vi "WaterFall.vi"() -> ()   [LabVIEW 2014]
uses:
  <vilib>/Simulation/Scripting/Companion Diagram/SimConfigNode/SimParams.ctl
  <vilib>/Simulation/Scripting/Companion Diagram/SimConfigNode/_simSolvers.ctl
  <vilib>/Simulation/Implementation/Shared/SIMSCR Execution Mode.ctl
  <vilib>/Simulation/Param Hierarchy/Typedefs/SIMPH Param Control Actions.ctl
  <vilib>/Simulation/Implementation/Shared/SIM limit type.ctl
  <vilib>/Simulation/Implementation/Shared/NILVSim_ParamChanged.vi
  <vilib>/Simulation/Implementation/Shared/NILVSIM_BeginStep.vi
  <vilib>/Simulation/DataSources/Implementation/NILVSim Step.llb/SIM Step (scalar).vi
  <vilib>/Simulation/Nonlinear/Implementation/NILVSim Switch.llb/SIM Switch (scalar).vi
  <vilib>/Simulation/DataSources/Implementation/NILVSim Pulse Generator.llb/SIM Pulse Generator (scalar).vi
  <vilib>/Simulation/ContinuousLinear/Implementation/NILVSim Transfer Function.llb/SIM Transfer Function Distributor (SISO).vi
  <vilib>/Simulation/ContinuousLinear/Implementation/NILVSim Integrator new.llb/SIM Integrator distributor (scalar).vi
  <vilib>/Simulation/ContinuousLinear/Implementation/NILVSim Derivative.llb/SIM derivative (scalar).vi
  <vilib>/Simulation/Nonlinear/Implementation/NILVSim Saturation.llb/SIM Saturation (scalar).vi
  <vilib>/Simulation/ContinuousLinear/Implementation/NILVSim Transport Delay.llb/SIM Transport Delay Distributor (scalar).vi
  <vilib>/Simulation/ContinuousLinear/Implementation/NILVSim Transport Delay.llb/SIM Transport Delay Collector (scalar).vi
  <vilib>/Simulation/ContinuousLinear/Implementation/NILVSim Integrator new.llb/SIM Integrator collector (scalar).vi
  <vilib>/Simulation/SignalDisplay/Implementation/NILVSim Time Waveform.llb/SIM Time Waveform (vector).vi
  <vilib>/Simulation/ContinuousLinear/Implementation/NILVSim Transfer Function.llb/SIM Transfer Function Collector (SISO).vi
  <vilib>/Simulation/Implementation/Shared/NILVSim_Manager.vi
  <vilib>/Utility/error.llb/Clear Errors.vi
  <vilib>/Simulation/Implementation/Shared/NILVSim_FinalizeModel.vi
  <vilib>/Simulation/Implementation/Shared/SIM Unbundle Sim Info.vi
  <vilib>/Simulation/Implementation/Shared/NILVSim_Initialize.vi
  <vilib>/Simulation/Utility/Implementation/NILVSim Get Time and IsAcceptedStep.vi
  <vilib>/Simulation/Implementation/Shared/SIMSH Read Queue.vi
  <vilib>/Simulation/Implementation/Shared/NILVSim_GetModelError.vi
  <vilib>/Simulation/Implementation/Shared/SIM Bundle Sim Info.vi
  <vilib>/Simulation/Scripting/Companion Diagram/SimConfigNode/SimDog.xnode
  <vilib>/Simulation/Implementation/XNodeFramework/SimXNode/SimX.xnode
  <vilib>/Simulation/ContinuousLinear/Implementation/NILVSim Integrator new.llb/SIM Integrator (scalar).vi
  <vilib>/Simulation/ContinuousLinear/Implementation/NILVSim Transport Delay.llb/SIM Transport Delay Indirect (scalar).vi
  <vilib>/Simulation/ContinuousLinear/Implementation/NILVSim Transfer Function.llb/SIM Transfer Function (SISO).vi
  <vilib>/Simulation/Implementation/Shared/NI_SIM_Implementation.lvlib
panel:
  in  "F1_0 2":dbl=1.0
  out "X 0":dbl caption="ISE 2"
  in  "tpm":dbl
  in  "Ttm":dbl
  in  "Kpm":dbl
  in  "Ks":dbl
  in  "tps":dbl
  out "Kcs":dbl
  out "Tis":dbl
  out "Kcm":dbl
  out "Tim":dbl
  out "Tdm":dbl
  in  "Incremento P1\nAmplitud":dbl=0.05
  out "DP1 Perturbacion":dbl caption="ISE 2"
  in  "Incremento P1\nduracion":dbl=10.0
  in  "Retardo en la \ntuberia":dbl=3.0
  in  "Fd Duraci—n\n perturbaci—n":dbl=10.0
  in  "1=ZN, 0=AMIGO":dbl
  out "Kc":dbl
  out "Ti":dbl
  out "Td":dbl
  in  "F1_0":dbl=1.0
  in  "H0":dbl=1.0
  in  "Href":dbl=1.0
  out "Fd Perturbacion":dbl caption="ISE 2"
  out "Tank  Cascade":dbl(slide) scale=0.0..4.0
  out "ISE 2":dbl
  out "ISE 1":dbl
  out "input flow":waveform(dbl)[](graph)
  in  "factor Kc":dbl=1.0
  in  "factor Td":dbl=1.0
  in  "Fd Amplitud\n perturbacion":dbl
  out "Td2":dbl
  out "Ti2":dbl
  out "Kc2":dbl
  out "Td1":dbl
  out "Ti1":dbl
  out "Kc1":dbl
  in  "tp":dbl=2.0
  in  "Tt":dbl=3.0
  in  "Kp":dbl=20.0
  out "ISE":waveform(dbl)[](graph)
  out "Tank B.R.C.":dbl(slide) scale=0.0..4.0
  in  "K1":dbl=1.0
  in  "A1":dbl=1.0
  in  "factor Ti":dbl=1.0
  out "Alturas":waveform(dbl)[](graph)
  # "Estudio del control en cascada"
  # "Altura de Referencia"
  # "PERTURBACIONES"
  # "SISTEMA"
  # "IDENTIFICACIÓN\nC.R.B."
  # "IDENTIF. \nESCLAVO"
  # "IDENTIF. \nMAESTRO"
  # "CONTROLADOR\nESCLAVO"
  # "CONTROLADOR\nMAESTRO"
  # "C.R.B"
  # "Z-N"
  # "AMIGO"
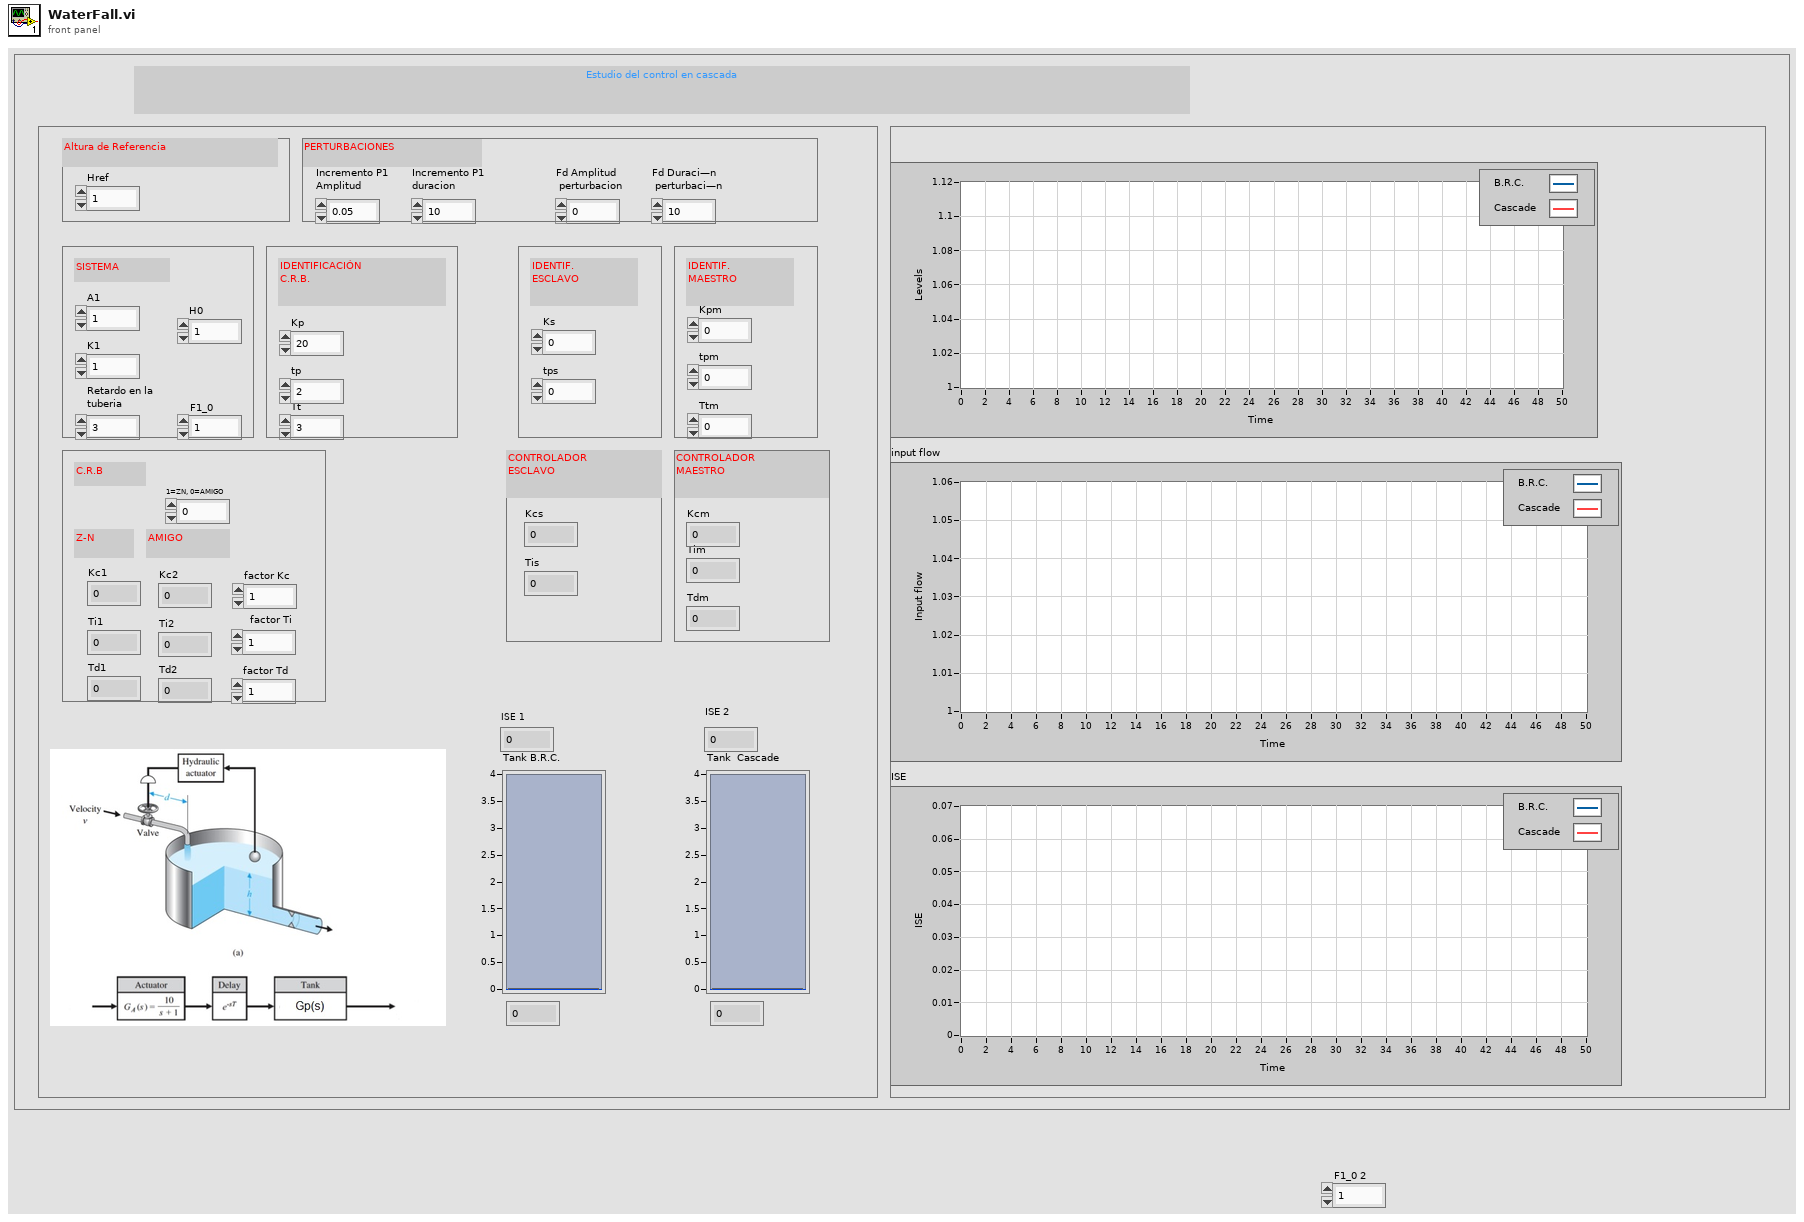
[diagram p1: front panel]
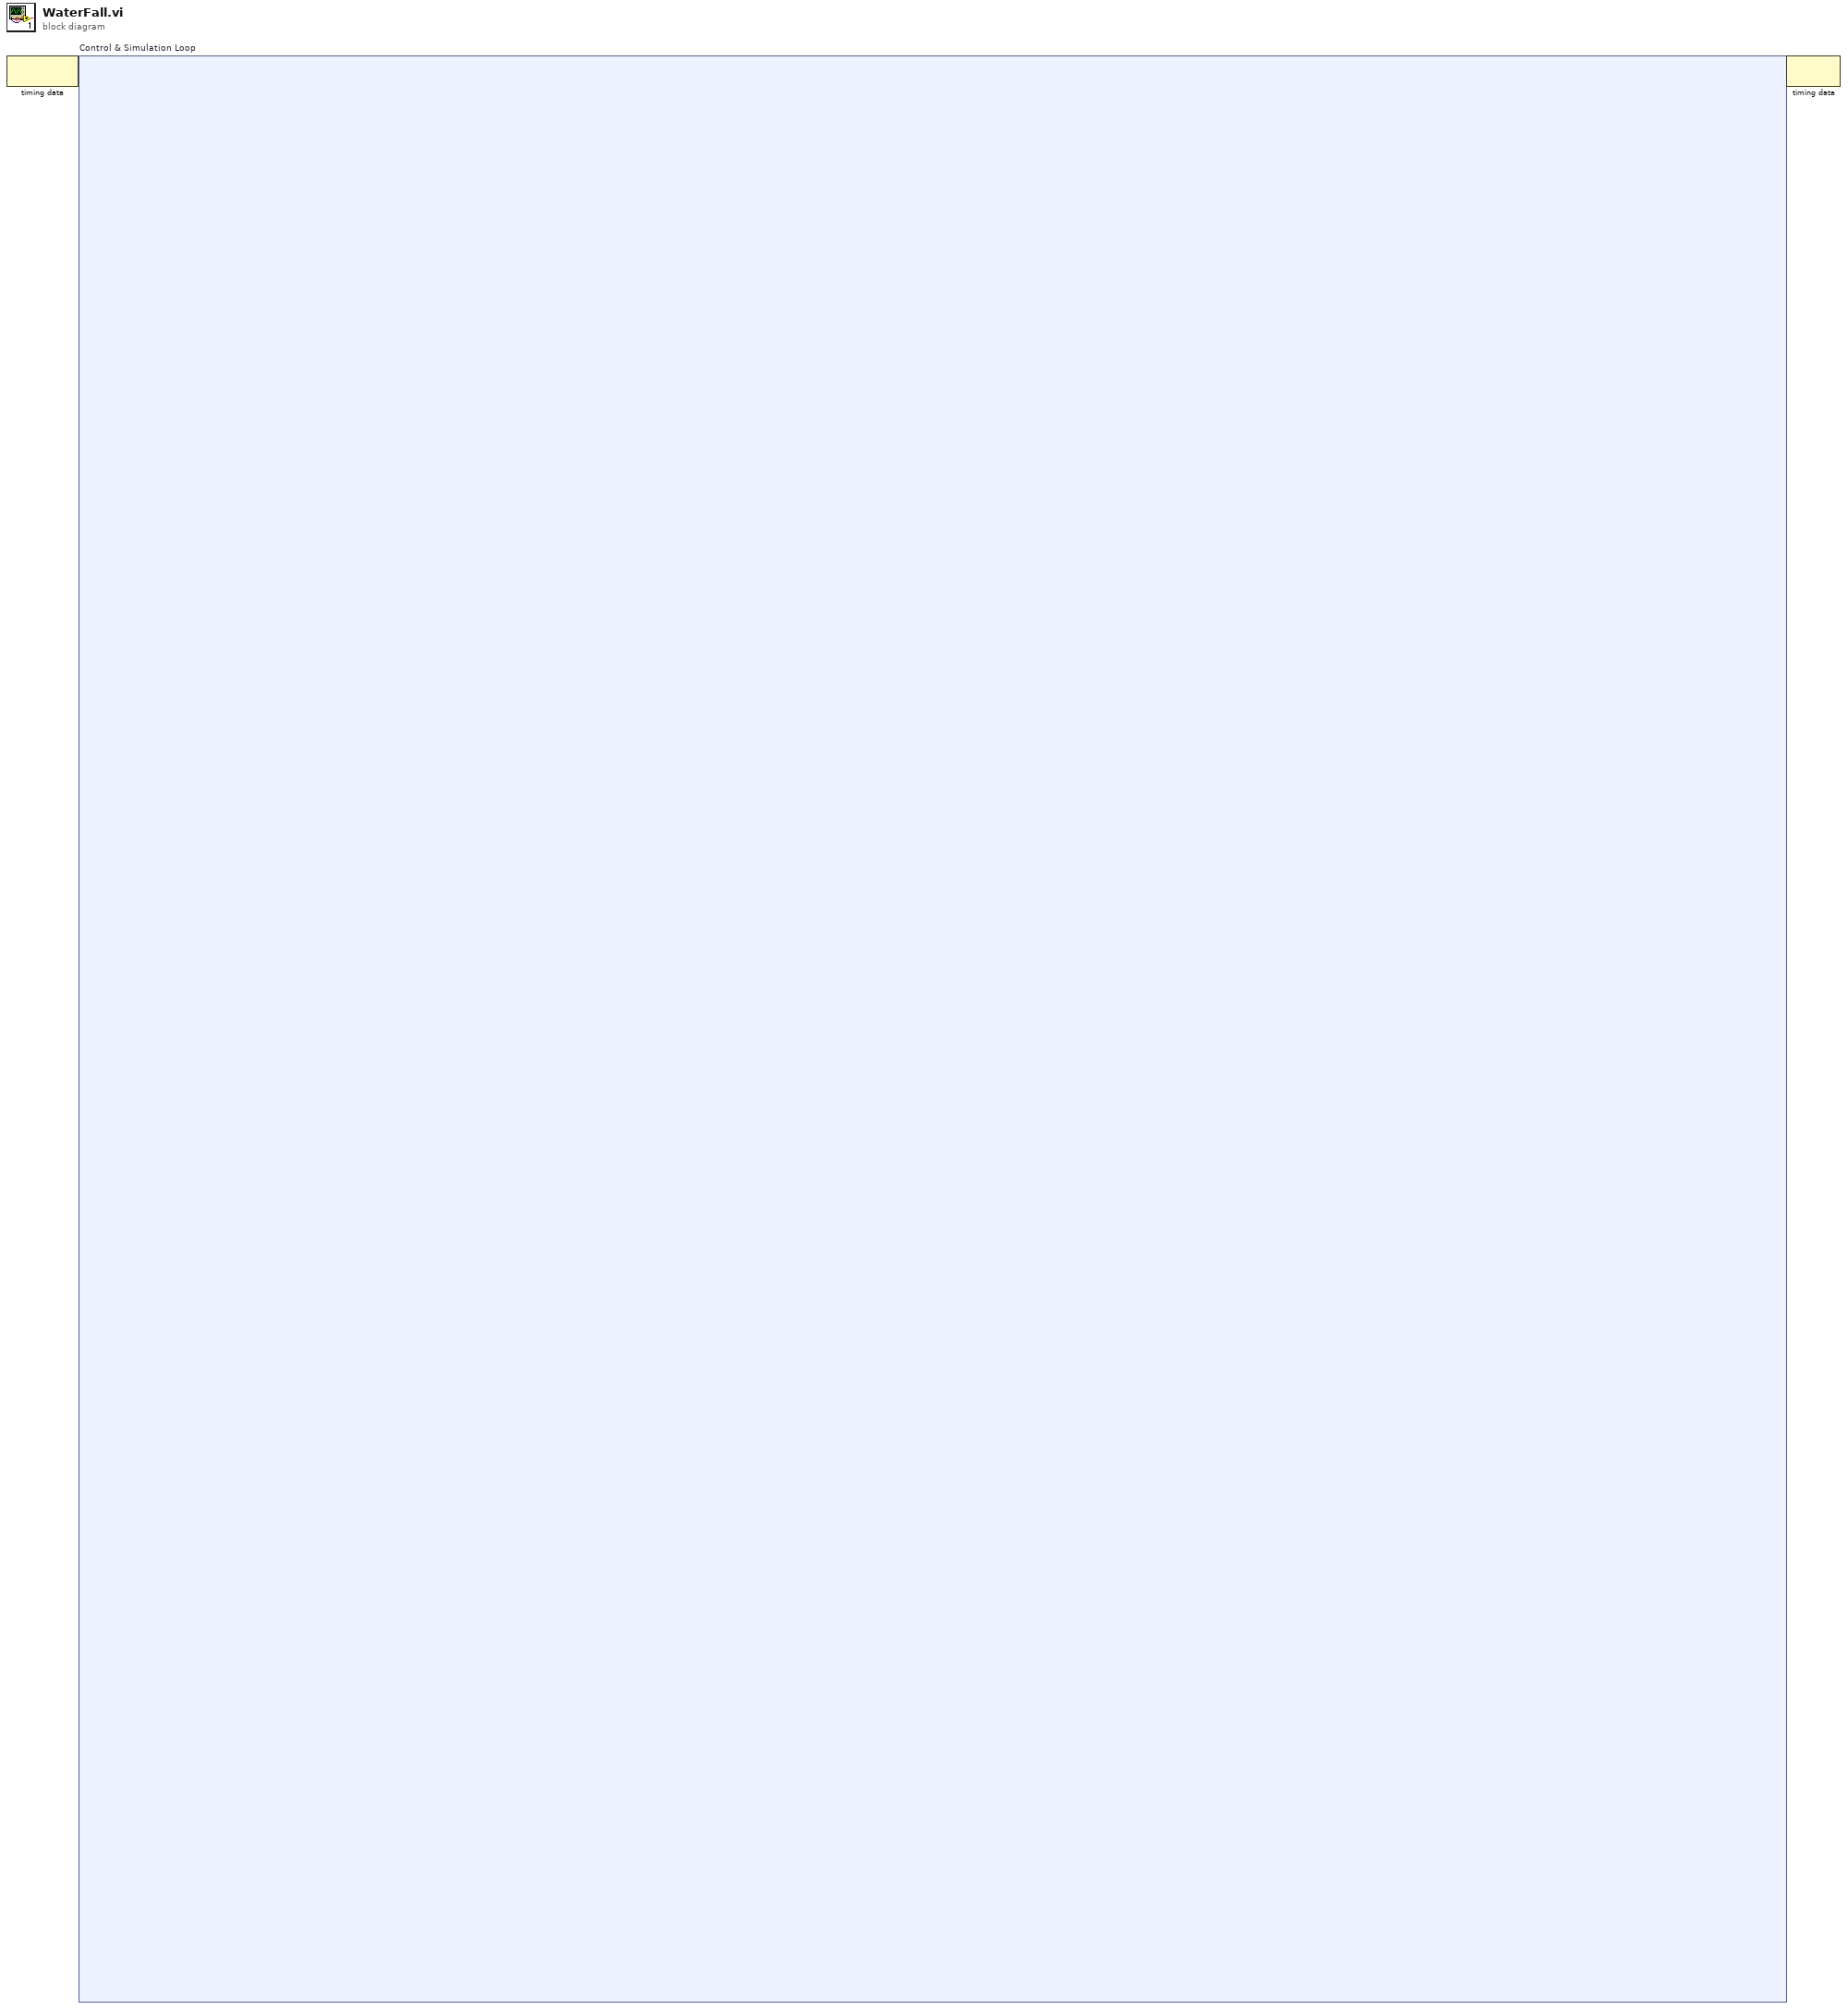
[diagram p0: block diagram]
diagram:
  n1 = node-c288() -> (w2:variant)  [unwired: 1 in]
  n2 = node-c254 "Control & Simulation Loop"(w2) -> (w1:variant)
  n3 = node-c288(w1) -> ()  [unwired: 1 out]
